vi "Init Analysis Graph.vi"(6 "Z Scale.Marker Values[]":cluster{"Numeric":dbl, "Numeric":u32}[](array[cluster]), 7 "Graphs":T1, 8 "error in":errorcluster, 9 "Shots":u32, 10 "Image Size":cluster{"Height":u32, "Width":u32}, 11 "Analysis Graph in":refnum<class "Graph with Analysis Controls.lvclass">) -> (0 "error out":errorcluster, 3 "Analysis Graph out":refnum<class "Graph with Analysis Controls.lvclass">)   [LabVIEW 2023, in "Graph with Analysis Controls.lvclass"]
uses:
  Graph with Analysis Controls.lvclass
  Graph with Analysis Controls.lvclass/Graph with Analysis Controls.ctl
  Series Graph/Graph with Series View.lvclass
  D:/git/Lock-In-Thermography-Graphs/source/Series Graph/Graph with Series View.lvclass
  D:/git/Lock-In-Thermography-Graphs/source/Detail Graph/Graph with Section Views.lvclass
  D:/git/Lock-In-Thermography-Graphs/source/Base Graph/Base Graph.lvclass
  D:/git/Lock-In-Thermography-Graphs/source/Analysis Graph/Graph with Analysis Controls.lvclass
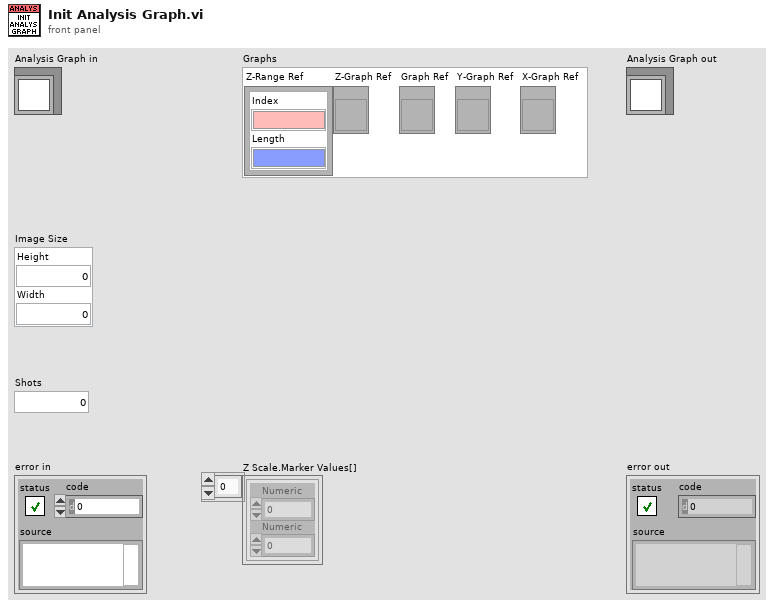
[diagram p1: front panel]
types:
  T1 = cluster{"Z-Range Ref":refnum<vi>, "Z-Graph Ref":refnum<vi>, "Graph Ref":refnum<vi>, "Y-Graph Ref":refnum<vi>, "X-Graph Ref":refnum<vi>}
  T2 = cluster{"Z-Graph Ref":refnum<vi>, "Graph Ref":refnum<vi>, "Y-Graph Ref":refnum<vi>, "X-Graph Ref":refnum<vi>}
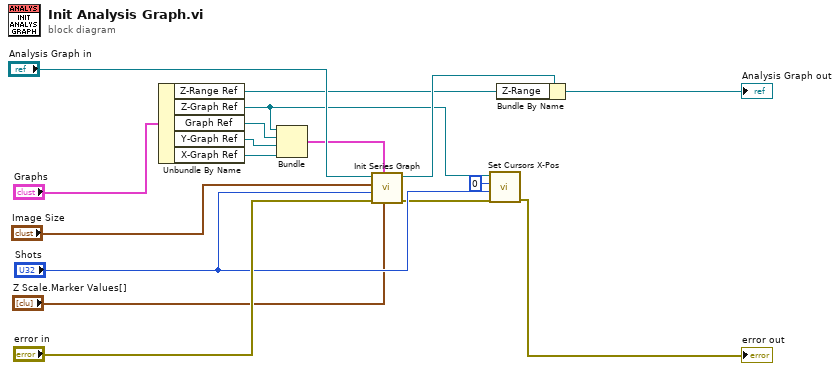
[diagram p0: block diagram]
diagram:
  n1 = Unbundle By Name("Graphs") -> ("Z-Range Ref"=w2:refnum<vi>, "Z-Graph Ref"=w1:refnum<vi>, "Graph Ref"=w9:refnum<vi>, "Y-Graph Ref"=w8:refnum<vi>, "X-Graph Ref"=w7:refnum<vi>)
  n2 = Bundle("Z-Graph Ref"=w1, "Graph Ref"=w9, "Y-Graph Ref"=w8, "X-Graph Ref"=w7) -> (w6:T2)  [unwired: 1 in]
  n3 = call "Init Series Graph.vi"("Z Scale.Marker Values[]"="Z Scale.Marker Values[]", "Graphs"=w6, "error in"="error in", "Shots"="Shots", "Image Size"="Image Size", "Series Graph in"="Analysis Graph in") -> ("error out"=w3:errorcluster, "Series Graph out"=w5:refnum<class "Graph with Analysis Controls.lvclass">)  [unwired: 4 in]
  n4 = call "Set Cursors X-Pos.vi"("error in"=w3, "length"="Shots", "index"=0, "WaveformGraph in"=w1) -> ("error out"=→"error out":errorcluster)  [unwired: 7 in]
  n5 = Bundle By Name(cluster=w5, "Z-Range"=w2) -> (→"Analysis Graph out":refnum<class "Graph with Analysis Controls.lvclass">)
